vi "PWM CAP Init.vi"(9 "TimePrecUs":u8, 10 "Channel":u8, 11 "DevHandle":i32) -> (3 "function return":i32)   [LabVIEW 2010, in "usb2pwm.lvlib"]
doc: "int WINAPI PWM_CAP_Init(int DevHandle, unsigned char Channel,unsigned char TimePrecUs);"
uses:
  usb2pwm.lvlib
  USB2XXX/trunk/USB2XXX/USB2XXX/vs2019/Release/USB2XXX.dll
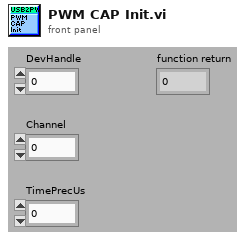
[diagram p1: front panel]
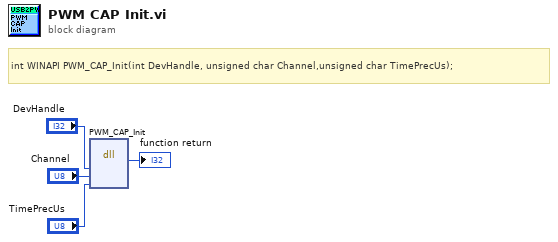
[diagram p0: block diagram]
diagram:
  # "int WINAPI PWM_CAP_Init(int DevHandle, unsigned char Channel,unsigned char TimePrecUs);"
  n1 = dll-call lib="E:/Projects/USB2XXX/trunk/USB2XXX/USB2XXX/vs2019/Release/USB2XXX.*" fn="PWM_CAP_Init"("DevHandle"="DevHandle", "Channel"="Channel", "TimePrecUs"="TimePrecUs") -> (→"function return":i32)  [unwired: 6 in, 2 out]
